vi "PH_AxisGUI_NF.ProcEvents.vi"(0 "i ref in":refnum<vi>, 5 "error in":errorcluster) -> (14 "i ref out":refnum<vi>, 19 "error out":errorcluster)   [LabVIEW 2014, in "PH_AxisGUI_NF.lvlib"]
doc: "This method is used to define the events the object will listen to. Add your own events here."
uses:
  PH_AxisGUI_NF.lvlib
  CS_Core/BaseProcess/BaseProcess.lvlib
  PH_Basics/PH_Common/PH_Common.lvlib
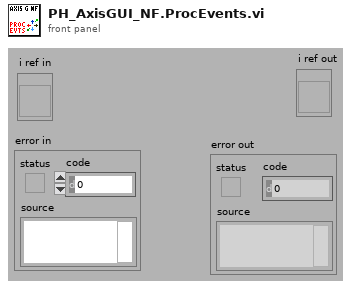
[diagram p1: front panel]
types:
  T1 = typedef "PH_AxisGUI_NF.lvlib/PH_AxisGUI_NF.i attribute.ctl" = cluster{"GUI Refs":cluster{"Delete":refnum<vi>, "Slide 0":refnum<vi>, "Slide 1":refnum<vi>, "Slide 2":refnum<vi>, "Instance Status":refnum<vi>, "Position":refnum<vi>, "Reset":refnum<vi>, "Goal":refnum<vi>, "Go":refnum<vi>}, "Instance":string, "Name Axis 0":string, "Name Axis 1":string, "Name Axis 2":string, "System":string, "Driver Type":T2, "Offset":i32, "Goal":i32}
  T2 = typedef "NF87XX.lvlib/NF87XX.driver Type.ctl" = enum16{"not defined", "3-ch open loop drv", "1-ch closed loop drv"}
  T3 = typedef "PH_Common.lvlib/PH_DIM.Event Declarer.ctl" = cluster{"Service Name":string, "Selector":string}
  T4 = typedef "BaseProcess.lvlib/BaseProcess.event definition.ctl" = cluster{"CAEEvtDef":T5, "Data Descriptor":T6}
  T5 = typedef "CAEObj.lvlib/CAEObj.event definition.ctl" = cluster{"URL":string, "enable":bool, "ignoreResID":bool}
  T6 = typedef "BaseProcess.lvlib/BaseProcess.descriptor string definition.ctl" = string
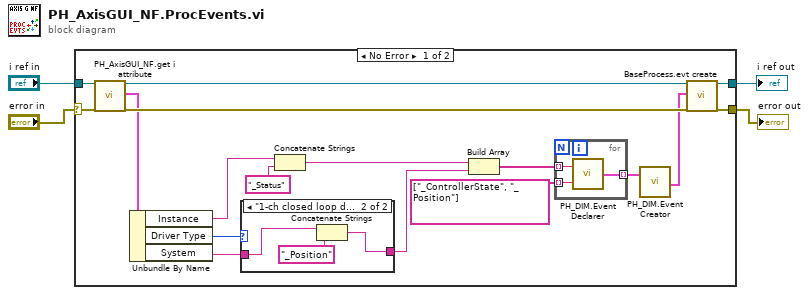
[diagram p0: block diagram]
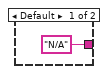
[diagram p2: hidden frame]
diagram:
  n1 = case shown="No Error" "error in" {
    selector: "error in" -> [w16 w29]
    tunnel: "i ref in" -> [w18 w30]
    tunnel: [w21 w30] -> w3
    tunnel: [w20 w29] -> w2
    frame No Error {
      n2 = call "PH_AxisGUI_NF.get i attribute.vi"("i ref in"=w18, "error in (no error)"=w16) -> ("i ref out"=w17:refnum<vi>, "i attribute"=w14:T1, "error out"=w15:errorcluster)  [unwired: 15 in]
      n3 = Unbundle By Name(w14) -> ("Instance"=w12:string, "Driver Type"=w11:T2, "System"=w10:string)
      n4 = case shown="\"1-ch closed loop drv\"" w11 {
        tunnel: w10 -> [_ w27]
        tunnel: ["N/A" w26] -> w9
        frame Default {
        }
        frame "1-ch closed loop drv" {
          n5 = Concatenate Strings(w27, "_Position" ("string")) -> (w26:string)
        }
      }
      n6 = Concatenate Strings(w12, "_Status" ("string")) -> (w13:string)
      n7 = Build Array(w13, w9) -> (w5:string[])
      n8 = for {
        tunnel: [w24] -> w8 mode=indexing
        tunnel: string[] ["_ControllerState", "_Position"] -> [w23] mode=indexing
        tunnel: w5 -> [w22] mode=indexing
        n9 = call "PH_DIM.Event Declarer.vi"("Selector"=w23, "Service Name"=w22) -> ("declared DIM Event"=w24:T3)
      }
      n10 = call "PH_DIM.Event Creator.vi"("Trendmessage Services"=w8) -> ("DIM Service Events"=w7:T4[])  [unwired: 18 in]
      n11 = call "BaseProcess.evt create.vi"("i ref in"=w17, "newEvents"=w7, "error in (no error)"=w15) -> ("i ref out"=w21:refnum<vi>, "error out"=w20:errorcluster)  [unwired: 13 in, 2 out]
    }
    frame Error {
    }
  }
  "i ref out" <- w3
  "error out" <- w2
